vi "XY图标尺字号自适应.vi"(6 "标尺字号":i16=5, 11 "XY图-引用":refnum<vi>) -> (0 "错误输出 2":errorcluster caption="错误输出")   [LabVIEW 2017]
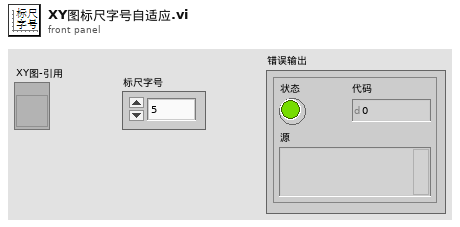
[diagram p1: front panel]
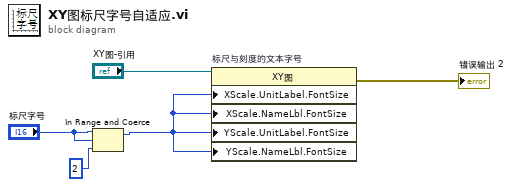
[diagram p0: block diagram]
diagram:
  n1 = In Range and Coerce(upper limit="标尺字号", x="标尺字号", lower limit=i16 2 ("下限")) -> (coerced(x)=w1:i16)  [unwired: 1 out]
  n2 = property on="标尺与刻度的文本字号" class="XY图"(reference="XY图-引用", "XScale.UnitLabel.FontSize"=w1, "XScale.NameLbl.FontSize"=w1, "YScale.UnitLabel.FontSize"=w1, "YScale.NameLbl.FontSize"=w1) -> (error out=→"错误输出 2":errorcluster)  [unwired: 1 in, 1 out]
